vi "ZCAN_Setcn.vi"(8 "error in (no error)":errorcluster caption="错误输入（无错误）", 9 "cn":string, 10 "channelIdx":u32, 11 "device_handle":u32) -> (0 "error out":errorcluster caption="错误输出")   [LabVIEW 2018]
doc: "该函数用于清除库接收缓冲区。"
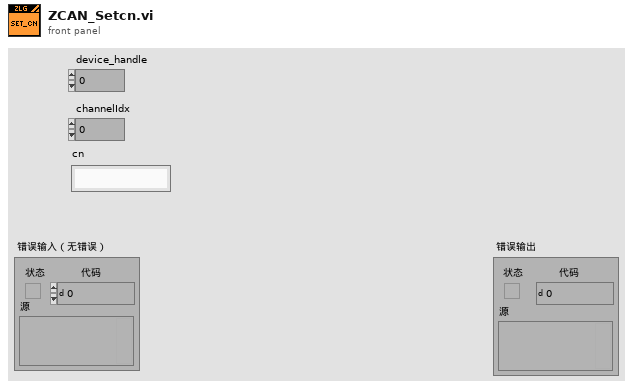
[diagram p1: front panel]
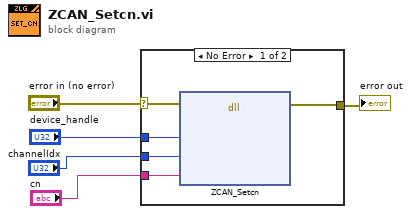
[diagram p0: block diagram]
diagram:
  n1 = case shown="No Error" "error in (no error)" {
    selector: "error in (no error)" -> [w9 w11]
    tunnel: [w6 w11] -> w4
    tunnel: "device_handle" -> [w10 _]
    tunnel: "channelIdx" -> [w8 _]
    tunnel: "cn" -> [w7 _]
    frame No Error {
      n2 = dll-call lib="PTH2kabs CUsersadminDesktopzlgcan_demo_20220516_2018版本zlgcan_demo_USBCANFDbinzlgcan_wrap.dll" fn="ZCAN_Setcn" ("ZCAN_StartCAN")(error in=w9, "device_handle"=w10, "channelIdx"=w8, "cn"=w7) -> (error out=w6:errorcluster)  [unwired: 6 in, 1 out]
    }
    frame Error {
    }
  }
  "error out" <- w4
